vi "Verify CLI STD ERR.vi"(8 "error in":errorcluster) -> (0 "error out":errorcluster)   [LabVIEW 2020, in "Caraya Extension Tests.lvclass"]
uses:
  Caraya Extension Tests.lvclass
  Caraya Extension Tests.lvclass/Caraya Extension Tests.ctl
  <vilib>/addons/_JKI Toolkits/Caraya/classes/Test/Test.lvclass
  Source/Extensions/Caraya.Extension/Caraya.Extension.lvlib
  Source/Approval Tests/Approval Tests.lvlib
  Source/Approval Tests/OS Strings.ctl
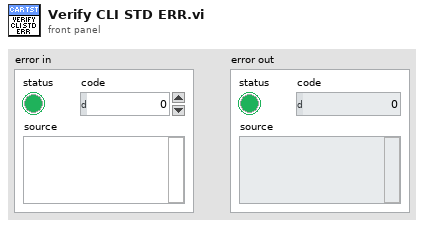
[diagram p1: front panel]
types:
  T1 = typedef "Approval Tests.lvlib/OS Strings.ctl" = cluster{"Windows":string, "Linux":string, "Mac":string}
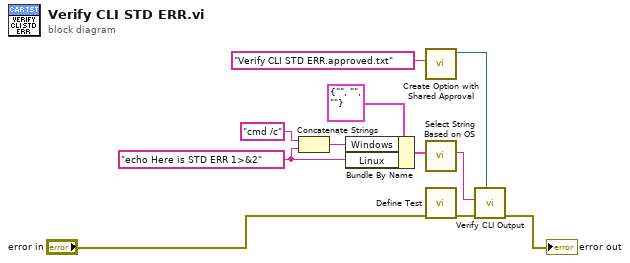
[diagram p0: block diagram]
diagram:
  w1 = "echo Here is STD ERR 1>&2" ("command line")
  n1 = Concatenate Strings("cmd /c" ("string"), w1) -> (w2:string)
  n2 = Bundle By Name(cluster=T1 {"Windows"="", "Linux"="", "Mac"=""} ("Strings"), "Windows"=w2, "Linux"=w1) -> (w3:T1)
  n3 = call "Create Option with Shared Approval.vi"("Filename"="Verify CLI STD ERR.approved.txt") -> ("Options outs"=w8:refnum<class "Options.lvclass">)  [unwired: 10 in]
  n4 = call "Select String Based on OS.vi"("Strings"=w3) -> ("Selection"=w6:string)  [unwired: 10 in]
  n5 = call <vilib>:"Define Test.vi"("error in (no error)"="error in") -> ("error out"=w9:errorcluster)  [unwired: 9 in, 1 out]
  n6 = call "Verify CLI Output.vi"("Options"=w8, "error in"=w9, "command line"=w6) -> ("error out"=→"error out":errorcluster)  [unwired: 7 in, 1 out]
